vi "SW_Load_settings_from_previous_experiments.vi"(0 "File to load data from":path, 2 "User Name":string="Researcher", 3 "error in (no error)":errorcluster) -> (6 "Settings cluster out":T1, 7 "IO parameters cluster":T2, 9 "Stimulus presets array":T3(array[cluster])=[{"Event type"=0, "Dur., s"=0.0, "Stim., s"=0.0, "Set/Clear"=FALSE, "TTL out N"=1, "Stim. has been set"=FALSE}, {"Event type"=0, "Dur., s"=0.0, "Stim., s"=0.0, "Set/Clear"=FALSE, "TTL out N"=1, "Stim. has been set"=FALSE}, {"Event type"=0, "Dur., s"=0.0, "Stim., s"=0.0, "Set/Clear"=FALSE, "TTL out N"=1, "Stim. has been set"=FALSE}, {"Event type"=0, "Dur., s"=0.0, "Stim., s"=0.0, "Set/Clear"=FALSE, "TTL out N"=1, "Stim. has been set"=FALSE}, {"Event type"=0, "Dur., s"=0.0, "Stim., s"=0.0, "Set/Clear"=FALSE, "TTL out N"=1, "Stim. has been set"=FALSE}, {"Event type"=0, "Dur., s"=0.0, "Stim., s"=0.0, "Set/Clear"=FALSE, "TTL out N"=1, "Stim. has been set"=FALSE}, {"Event type"=0, "Dur., s"=0.0, "Stim., s"=0.0, "Set/Clear"=FALSE, "TTL out N"=1, "Stim. has been set"=FALSE}, {"Event type"=0, "Dur., s"=0.0, "Stim., s"=0.0, "Set/Clear"=FALSE, "TTL out N"=1, "Stim. has been set"=FALSE}, {"Event type"=0, "Dur., s"=0.0, "Stim., s"=0.0, "Set/Clear"=FALSE, "TTL out N"=1, "Stim. has been set"=FALSE}, {"Event type"=0, "Dur., s"=0.0, "Stim., s"=0.0, "Set/Clear"=FALSE, "TTL out N"=1, "Stim. has been set"=FALSE}, {"Event type"=0, "Dur., s"=0.0, "Stim., s"=0.0, "Set/Clear"=FALSE, "TTL out N"=1, "Stim. has been set"=FALSE}, {"Event type"=0, "Dur., s"=0.0, "Stim., s"=0.0, "Set/Clear"=FALSE, "TTL out N"=1, "Stim. has been set"=FALSE}, {"Event type"=0, "Dur., s"=0.0, "Stim., s"=0.0, "Set/Clear"=FALSE, "TTL out N"=1, "Stim. has been set"=FALSE}, {"Event type"=0, "Dur., s"=0.0, "Stim., s"=0.0, "Set/Clear"=FALSE, "TTL out N"=1, "Stim. has been set"=FALSE}] {"Event type" items=["Stay for N seconds"]; "TTL out N" items=["1"=1, "2"=2, "1+2"=3]}, 10 "error out":errorcluster={"status"=TRUE, "code"=1, "source"="Dequeue Element in NI_LVConfig.lvlib:Read Value Without Comment.vi->NI_LVConfig.lvlib:Read Key (I32).vi->SW_Load_settings_to_main_tab.vi"})   [LabVIEW 2016]
uses:
  <vilib>/Utility/config.llb/Config Data RefNum.ctl
  <vilib>/Utility/config.llb/NI_LVConfig.lvlib
panel:
  out "Author's name":string
  out "Settings loaded OK (TDMS)":bool
  out "Data filtering":u16
  out "\"Stop at\" enabled":bool
  out "Name prefix":string
  out "Stop at":dbl
  out "Offset H.":dbl
  out "Twisted neck":bool
  out "Vertical offset":dbl
  out "Bridge swap?":bool
  out "VISA resource name":string
  out "Cage diameter, mm":i32=180
  out "Border segments starting angle":i32
  out "Midfield segments starting angle":i32
  out "Midfield segments outer radius, mm":i32=60
  out "Center segment outer radius, mm":i32=30
  out "Amount of border segments":i32=8
  out "Amount of midfield segments":i32=4
  out "Refnum out":T4
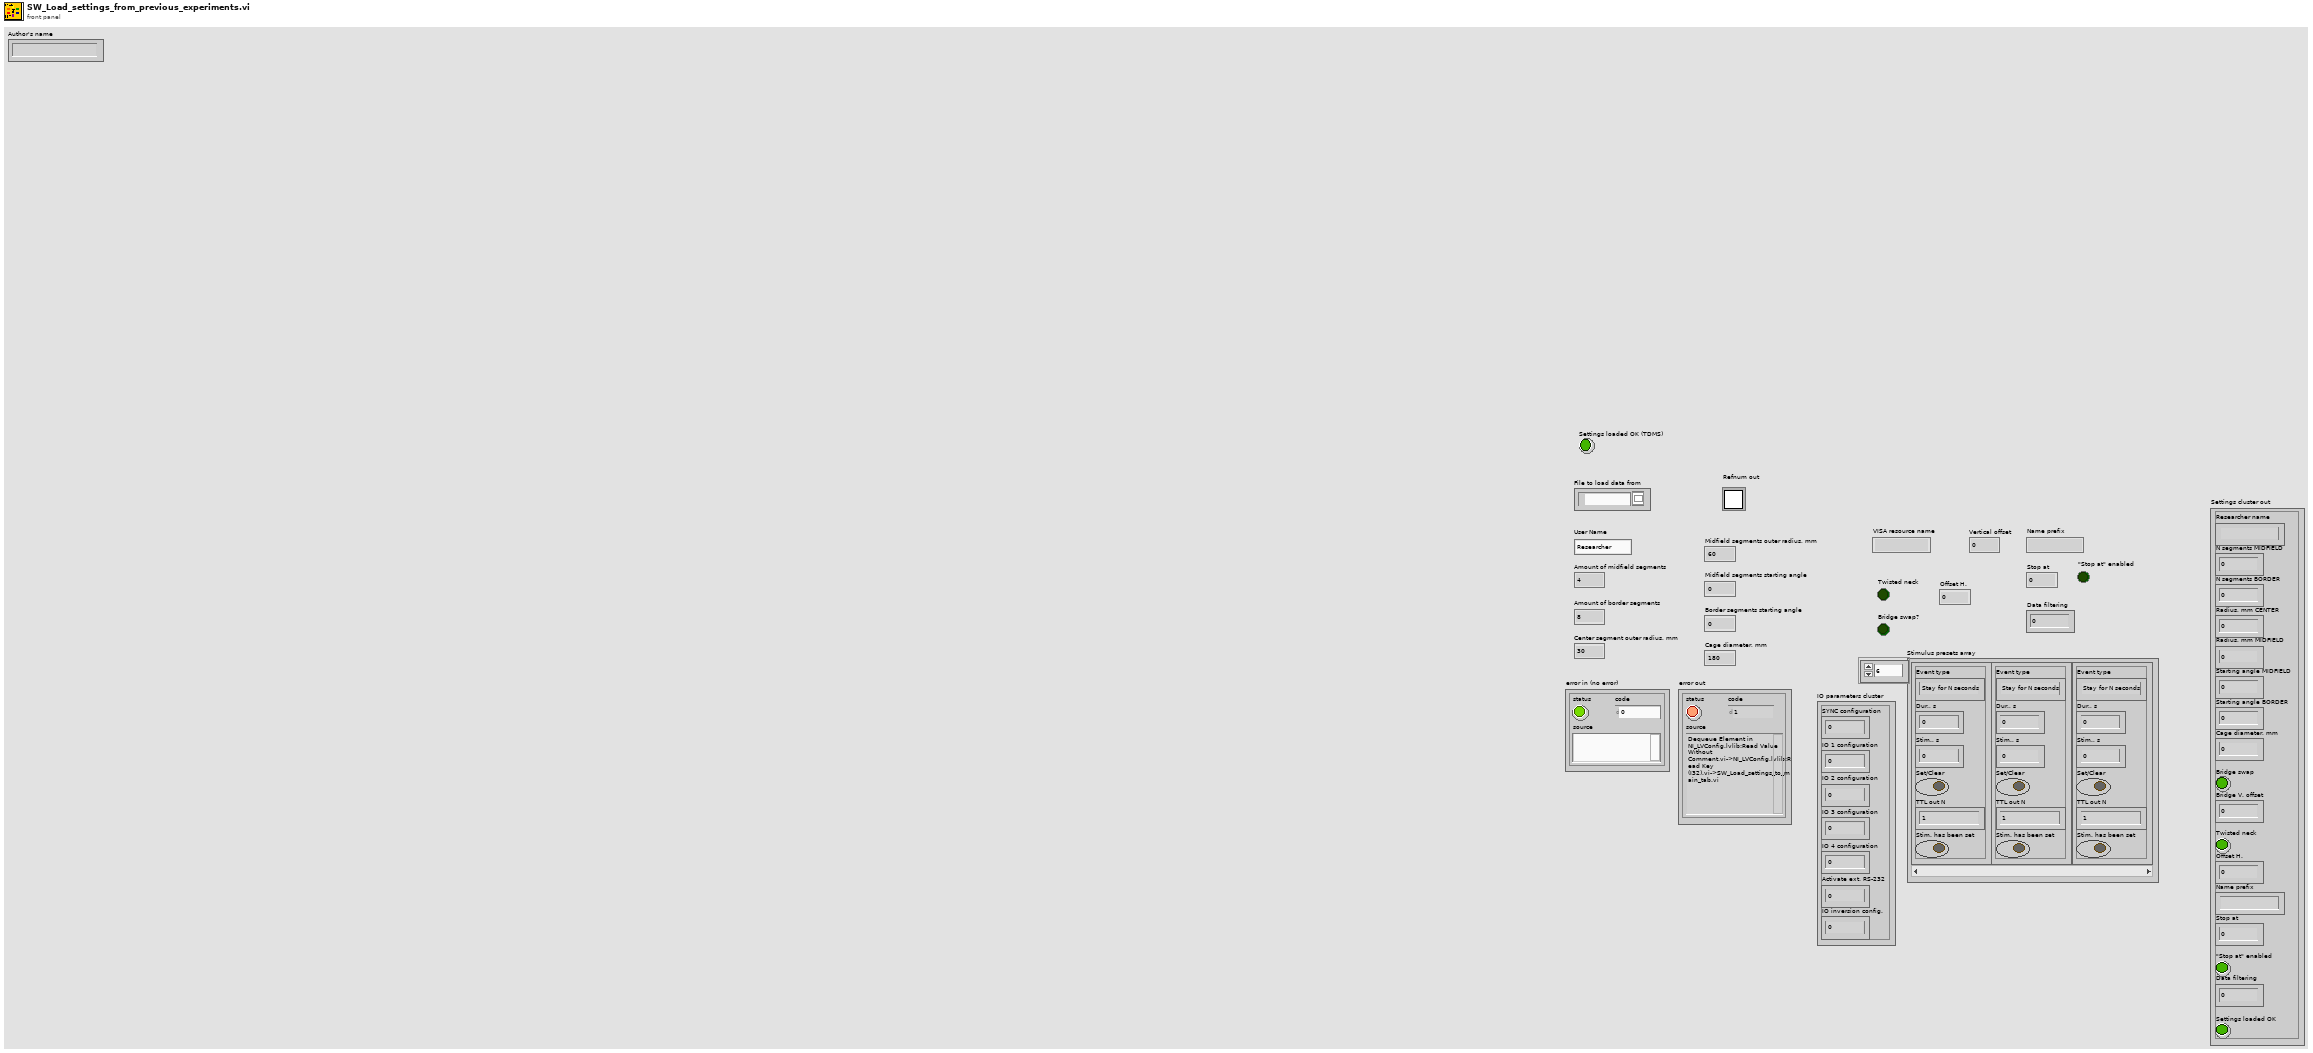
[diagram p1: front panel]
types:
  T1 = cluster{"Researcher name":string, "N segments MIDFIELD":u8, "N segments BORDER":u8, "Radius, mm CENTER":u16, "Radius, mm MIDFIELD":u16, "Starting angle MIDFIELD":i16, "Starting angle BORDER":i16, "Cage diameter, mm":u16, "Bridge swap":bool, "Bridge V. offset":sgl, "Twisted neck":bool, "Offset H.":sgl, "Name prefix":string, "Stop at":dbl, "\"Stop at\" enabled":bool, "Data filtering":u16, "Settings loaded OK":bool}
  T2 = cluster{"SYNC configuration":u16, "IO 1 configuration":u16, "IO 2 configuration":u16, "IO 3 configuration":u16, "IO 4 configuration":u16, "Activate ext. RS-232":u16, "IO inversion config.":u16}
  T3 = cluster{"Event type":u16, "Dur., s":sgl, "Stim., s":sgl, "Set/Clear":bool, "TTL out N":u16, "Stim. has been set":bool}[]
  T4 = typedef "NI_LVConfig.lvlib/Config Data RefNum.ctl" = refnum<k1>
  T5 = cluster{"N segments BORDER":u8, "Starting angle BORDER":i16, "N segments MIDFIELD":u8, "Starting angle MIDFIELD":i16, "Radius, mm MIDFIELD":u16, "Amount of central segments":u8, "Radius, mm CENTER":u16, "Bridge swap":bool, "Bridge V. offset":sgl, "Twisted neck":bool, "Offset H.":sgl, "Zones configuration":string[], "IO parameters string":string, "Cage diameter, mm":u16, "Name prefix":string, "Stop at":dbl, "\"Stop at\" enabled":bool, "Data filtering":u16}
  T6 = enum16{"big-endian, network order", "native, host order", "little-endian"}
  T7 = enum16{"open", "open or create", "create or replace", "create", "open (read-only)"}
  T8 = cluster{"Event type":u16, "Time, s":sgl, "Stimulus, s":sgl, "Set/Clear":bool, "TTL out":u16, "Stim. has been set":bool}
  T9 = cluster{"Event type":u16, "Cond., s":sgl, "Stim., s":sgl, "Set/Clear":bool, "TTL out N":u16, "Stim. has been set":bool}
  T10 = cluster{"array[0]":u16, "array[1]":u16, "array[2]":u16, "array[3]":u16, "array[4]":u16, "array[5]":u16, "array[6]":u16, "array[7]":u16, "array[8]":u16}
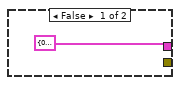
[diagram p2: hidden frame]
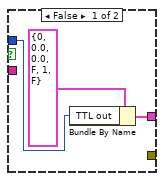
[diagram p10: hidden frame]
diagram:
  n1 = Path To String(path="File to load data from") -> (string=w13:string)
  n2 = To Lower Case(string=w13) -> (all lower case string=w12:string)
  n3 = Reverse String(1:w12) -> (0:w11:string)
  n4 = Search/Split String(string=w11, search string/char (-)=".") -> (substring before match=w9:string)  [unwired: 1 in, 2 out]
  n5 = Reverse String(1:w9) -> (0:w6:string)
  n6 = case shown="\"tdms\", Default" w6 {
    tunnel: [w30 w118] -> w8
    tunnel: [w49 w117] -> w7
    tunnel: "User Name" -> [_ w100]
    tunnel: "File to load data from" -> [w51 w116]
    tunnel: "error in (no error)" -> [w52 w114]
    tunnel: [w50 w112] -> w2
    tunnel: [w14 w111] -> w1
    frame "tdms", Default {
      n7 = TDMS Open(5:FALSE ("create index file? (T)"), 6:TRUE ("disable buffering? (T)"), 7:enum16{"1.0", "2.0"}."2.0" ("file format version (2.0)"), 8:w52, 9:T6."little-endian" ("byte order (2:little-endian)"), 10:T7."open (read-only)" ("operation (0:open)"), 11:w51) -> (0:w66:errorcluster, 3:w67:refnum<k34>)
      n8 = TDMS Get Properties(5:"", 7:"Description" ("property name"), 8:w66, 11:w67) -> (0:w62:errorcluster, 3:w61:refnum<k34>, 4:w63:string, 6:w56:bool)  [unwired: 2 in, 2 out]
      n9 = Unflatten From JSON(JSON string=w63, type and defaults=T5 {"N segments BORDER"=0, "Starting angle BORDER"=0, "N segments MIDFIELD"=0, "Starting angle MIDFIELD"=0, "Radius, mm MIDFIELD"=0, "Amount of central segments"=0, "Radius, mm CENTER"=0, "Bridge swap"=FALSE, "Bridge V. offset"=0.0, "Twisted neck"=FALSE, "Offset H."=0.0, "Zones configuration"=[], "IO parameters string"="[12,1,1,0,0,0]", "Cage diameter, mm"=180, "Name prefix"="SavedTrack", "Stop at"=0.0, "\"Stop at\" enabled"=FALSE, "Data filtering"=5} ("Parameters"), error in (no error)=w62) -> (value=w57:T5, error out=w58:errorcluster)  [unwired: 4 in]
      n10 = TDMS Get Properties(5:"", 7:"Author" ("property name"), 8:w58, 11:w61) -> (0:w27:errorcluster, 4:w47:string, 6:w55:bool)  [unwired: 2 in, 3 out]
      "Author's name" <- w47
      n11 = Unbundle By Name(w57) -> ("N segments MIDFIELD"=w46:u8, "N segments BORDER"=w44:u8, "Radius, mm CENTER"=w43:u16, "Radius, mm MIDFIELD"=w42:u16, "Starting angle MIDFIELD"=w41:i16, "Starting angle BORDER"=w40:i16, "Bridge V. offset"=w37:sgl, "Bridge swap"=w38:bool, "Cage diameter, mm"=w39:u16, "Zones configuration"=w54:string[], "Twisted neck"=w36:bool, "Offset H."=w35:sgl, "Name prefix"=w34:string, "Stop at"=w33:dbl, "\"Stop at\" enabled"=w32:bool, "Data filtering"=w31:u16, "IO parameters string"=w28:string)
      n12 = And(x=w56, y=w55) -> (x .and. y?=w45:bool)
      "Settings loaded OK (TDMS)" <- w45
      n13 = Bundle By Name(cluster=T1 {"Researcher name"="Researcher", "N segments MIDFIELD"=3, "N segments BORDER"=7, "Radius, mm CENTER"=30, "Radius, mm MIDFIELD"=75, "Starting angle MIDFIELD"=0, "Starting angle BORDER"=0, "Cage diameter, mm"=180, "Bridge swap"=FALSE, "Bridge V. offset"=0.0, "Twisted neck"=FALSE, "Offset H."=0.0, "Name prefix"="SavedTrack", "Stop at"=0.0, "\"Stop at\" enabled"=FALSE, "Data filtering"=5, "Settings loaded OK"=FALSE} ("Settings cluster out"), "Researcher name"=w47, "N segments MIDFIELD"=w46, "N segments BORDER"=w44, "Radius, mm CENTER"=w43, "Radius, mm MIDFIELD"=w42, "Starting angle MIDFIELD"=w41, "Starting angle BORDER"=w40, "Cage diameter, mm"=w39, "Bridge swap"=w38, "Bridge V. offset"=w37, "Twisted neck"=w36, "Offset H."=w35, "Name prefix"=w34, "Stop at"=w33, "\"Stop at\" enabled"=w32, "Data filtering"=w31, "Settings loaded OK"=w45) -> (w30:T1)
      n14 = Unflatten From JSON(JSON string=w28, type and defaults=u16[] [] ("array"), error in (no error)=w27) -> (value=w15:u16[], error out=w26:errorcluster)  [unwired: 4 in]
      n15 = Array To Cluster(array=w15) -> (cluster=w23:T10)
      n16 = Unbundle(w23) -> ("array[0]"=w22:u16, "array[1]"=w21:u16, "array[2]"=w20:u16, "array[3]"=w19:u16, "array[4]"=w18:u16, "array[5]"=w17:u16, "array[6]"=w16:u16)  [unwired: 2 out]
      n17 = Bundle By Name(cluster=T2 {"SYNC configuration"=12, "IO 1 configuration"=1, "IO 2 configuration"=1, "IO 3 configuration"=0, "IO 4 configuration"=0, "Activate ext. RS-232"=0, "IO inversion config."=0} ("Sync parameters cluster output"), "SYNC configuration"=w22, "IO 1 configuration"=w21, "IO 2 configuration"=w20, "IO 3 configuration"=w19, "IO 4 configuration"=w18, "Activate ext. RS-232"=w17, "IO inversion config."=w16) -> (w14:T2)
      n18 = for {
        N: 14 -> [_]
        tunnel: w26 -> [w77]
        tunnel: [w79] -> w50
        tunnel: [w80] -> w49 mode=indexing
        tunnel: w54 -> [w75]
        i -> [w76]
        n19 = for {
          tunnel: w75 -> [w91] mode=indexing
          tunnel: w76 -> [w85]
          tunnel: [w84] -> w74
          tunnel: [w83] -> w73
          stop <- w84 stop-if-true
          n20 = Search/Split String(string=w91, search string/char (-)=":") -> (substring before match=w89:string, match + rest of string=w82:string)  [unwired: 1 in, 1 out]
          n21 = String Subset(string=w82, offset (0)=2) -> (substring=w83:string)  [unwired: 1 in]
          n22 = Scan From String(format string="%u", input string=w89, initial scan location=u32 4) -> (output 1=w86:u32)  [unwired: 2 in, 3 out]
          n23 = Equal?(x=w85, y=w86) -> (x = y?=w84:bool)
        }
        n24 = case shown="True" w74 {
          tunnel: w73 -> [_ w96]
          tunnel: [T8 {"Event type"=0, "Time, s"=0.0, "Stimulus, s"=0.0, "Set/Clear"=FALSE, "TTL out"=1, "Stim. has been set"=FALSE} ("Cluster of the stimuls settings") w95] -> w80
          tunnel: [_ w94] -> w78
          frame False {
          }
          frame True {
            n25 = Unflatten From JSON(JSON string=w96, type and defaults=T8 {"Event type"=0, "Time, s"=0.0, "Stimulus, s"=0.0, "Set/Clear"=FALSE, "TTL out"=1, "Stim. has been set"=FALSE} ("Cluster of the stimuls settings")) -> (value=w95:T8, error out=w94:errorcluster)  [unwired: 5 in]
          }
        }
        n26 = Merge Errors(w78, w77) -> (w79:errorcluster)
      }
    }
    frame "trset" {
      w109 = "Data filtering" ("key")
      w140 = "\"Stop at\" enabled"
      w149 = "Stop at" ("key")
      w144 = "SavedTrack" ("default value")
      w152 = "Name prefix"
      w162 = "Offset H." ("key")
      w168 = "Twisted neck"
      w201 = "Bridge offset" ("key")
      w209 = "Bridge swap?"
      w218 = "Cage diameter, mm" ("key")
      w229 = "Border segments starting angle" ("key")
      w230 = "Midfield segments starting angle" ("key")
      w242 = "Midfield segments outer radius, mm" ("key")
      w245 = "Center segment outer radius, mm" ("key")
      w251 = "Amount of border segments" ("key")
      w260 = "Amount of midfield segments" ("key")
      n27 = call <vilib>:"Open Config Data.vi"("error in (no error)"=w114, "configuration file path"=w116) -> ("error out"=w113:errorcluster, "refnum"=w115:T4)  [unwired: 7 in, 1 out]
      n28 = call <vilib>:"Read Key (I32).vi"("section"=w100, "error in (no error)"=w113, "default value"=4, "key"=w260, "refnum"=w115) -> ("error out"=w258:errorcluster, "value"=w132:i32, "found?"=w261:bool)  [unwired: 3 in, 1 out]
      "Amount of midfield segments" <- w132
      n29 = case shown="False" w261 {
        tunnel: w100 -> [w428 _]
        tunnel: w115 -> [w429 w431]
        tunnel: w260 -> [w427 _]
        tunnel: w132 -> [w426 _]
        tunnel: w258 -> [w425 w430]
        tunnel: [w424 w430] -> w255
        tunnel: [w423 w431] -> w257
        frame False {
          n30 = call <vilib>:"Write Key (I32).vi"("section"=w428, "error in (no error)"=w425, "value"=w426, "key"=w427, "refnum"=w429) -> ("error out"=w424:errorcluster, "refnum out"=w423:T4)  [unwired: 4 in, 1 out]
        }
        frame True {
        }
      }
      n31 = call <vilib>:"Read Key (I32).vi"("section"=w100, "error in (no error)"=w255, "default value"=8, "key"=w251, "refnum"=w257) -> ("error out"=w252:errorcluster, "value"=w131:i32, "found?"=w253:bool, "refnum out"=w254:T4)  [unwired: 3 in]
      "Amount of border segments" <- w131
      n32 = case shown="False" w253 {
        tunnel: w100 -> [w419 _]
        tunnel: w254 -> [w420 w422]
        tunnel: w251 -> [w418 _]
        tunnel: w131 -> [w417 _]
        tunnel: w252 -> [w416 w421]
        tunnel: [w415 w421] -> w247
        tunnel: [w414 w422] -> w246
        frame False {
          n33 = call <vilib>:"Write Key (I32).vi"("section"=w419, "error in (no error)"=w416, "value"=w417, "key"=w418, "refnum"=w420) -> ("error out"=w415:errorcluster, "refnum out"=w414:T4)  [unwired: 4 in, 1 out]
        }
        frame True {
        }
      }
      n34 = call <vilib>:"Read Key (I32).vi"("section"=w100, "error in (no error)"=w247, "default value"=30, "key"=w245, "refnum"=w246) -> ("error out"=w250:errorcluster, "value"=w130:i32, "found?"=w249:bool, "refnum out"=w248:T4)  [unwired: 3 in]
      "Center segment outer radius, mm" <- w130
      n35 = case shown="False" w249 {
        tunnel: w100 -> [w410 _]
        tunnel: w248 -> [w411 w413]
        tunnel: w245 -> [w409 _]
        tunnel: w130 -> [w408 _]
        tunnel: w250 -> [w407 w412]
        tunnel: [w406 w412] -> w238
        tunnel: [w405 w413] -> w237
        frame False {
          n36 = call <vilib>:"Write Key (I32).vi"("section"=w410, "error in (no error)"=w407, "value"=w408, "key"=w409, "refnum"=w411) -> ("error out"=w406:errorcluster, "refnum out"=w405:T4)  [unwired: 4 in, 1 out]
        }
        frame True {
        }
      }
      n37 = call <vilib>:"Read Key (I32).vi"("section"=w100, "error in (no error)"=w238, "default value"=60, "key"=w242, "refnum"=w237) -> ("error out"=w239:errorcluster, "value"=w129:i32, "found?"=w240:bool, "refnum out"=w241:T4)  [unwired: 3 in]
      "Midfield segments outer radius, mm" <- w129
      n38 = case shown="False" w240 {
        tunnel: w100 -> [w401 _]
        tunnel: w241 -> [w402 w404]
        tunnel: w242 -> [w400 _]
        tunnel: w129 -> [w399 _]
        tunnel: w239 -> [w398 w403]
        tunnel: [w397 w403] -> w232
        tunnel: [w396 w404] -> w231
        frame False {
          n39 = call <vilib>:"Write Key (I32).vi"("section"=w401, "error in (no error)"=w398, "value"=w399, "key"=w400, "refnum"=w402) -> ("error out"=w397:errorcluster, "refnum out"=w396:T4)  [unwired: 4 in, 1 out]
        }
        frame True {
        }
      }
      n40 = call <vilib>:"Read Key (I32).vi"("section"=w100, "error in (no error)"=w232, "default value"=-90, "key"=w230, "refnum"=w231) -> ("error out"=w236:errorcluster, "value"=w128:i32, "found?"=w235:bool, "refnum out"=w234:T4)  [unwired: 3 in]
      "Midfield segments starting angle" <- w128
      n41 = case shown="False" w235 {
        tunnel: w100 -> [w392 _]
        tunnel: w234 -> [w393 w395]
        tunnel: w230 -> [w391 _]
        tunnel: w128 -> [w390 _]
        tunnel: w236 -> [w389 w394]
        tunnel: [w388 w394] -> w223
        tunnel: [w387 w395] -> w224
        frame False {
          n42 = call <vilib>:"Write Key (I32).vi"("section"=w392, "error in (no error)"=w389, "value"=w390, "key"=w391, "refnum"=w393) -> ("error out"=w388:errorcluster, "refnum out"=w387:T4)  [unwired: 4 in, 1 out]
        }
        frame True {
        }
      }
      n43 = call <vilib>:"Read Key (I32).vi"("section"=w100, "error in (no error)"=w223, "default value"=90, "key"=w229, "refnum"=w224) -> ("error out"=w225:errorcluster, "value"=w127:i32, "found?"=w226:bool, "refnum out"=w227:T4)  [unwired: 3 in]
      "Border segments starting angle" <- w127
      n44 = case shown="False" w226 {
        tunnel: w100 -> [w383 _]
        tunnel: w227 -> [w384 w386]
        tunnel: w229 -> [w382 _]
        tunnel: w127 -> [w381 _]
        tunnel: w225 -> [w380 w385]
        tunnel: [w379 w385] -> w216
        tunnel: [w378 w386] -> w217
        frame False {
          n45 = call <vilib>:"Write Key (I32).vi"("section"=w383, "error in (no error)"=w380, "value"=w381, "key"=w382, "refnum"=w384) -> ("error out"=w379:errorcluster, "refnum out"=w378:T4)  [unwired: 4 in, 1 out]
        }
        frame True {
        }
      }
      n46 = call <vilib>:"Read Key (I32).vi"("section"=w100, "error in (no error)"=w216, "default value"=180, "key"=w218, "refnum"=w217) -> ("error out"=w222:errorcluster, "value"=w126:i32, "found?"=w221:bool, "refnum out"=w220:T4)  [unwired: 3 in]
      "Cage diameter, mm" <- w126
      n47 = case shown="False" w221 {
        tunnel: w100 -> [w374 _]
        tunnel: w220 -> [w375 w377]
        tunnel: w218 -> [w373 _]
        tunnel: w126 -> [w372 _]
        tunnel: w222 -> [w371 w376]
        tunnel: [w370 w376] -> w104
        tunnel: [w369 w377] -> w102
        frame False {
          n48 = call <vilib>:"Write Key (I32).vi"("section"=w374, "error in (no error)"=w371, "value"=w372, "key"=w373, "refnum"=w375) -> ("error out"=w370:errorcluster, "refnum out"=w369:T4)  [unwired: 4 in, 1 out]
        }
        frame True {
        }
      }
      n49 = call <vilib>:"Read Key (U32).vi"("section"=w100, "error in (no error)"=w104, "default value"=5, "key"=w109, "refnum"=w102) -> ("error out"=w105:errorcluster, "value"=w110:u32, "found?"=w106:bool, "refnum out"=w107:T4)  [unwired: 3 in]
      n50 = To Unsigned Word Integer(number=w110) -> (unsigned 16bit integer=w97:u16)
      "Data filtering" <- w97
      n51 = case shown="False" w106 {
        tunnel: w100 -> [w267 _]
        tunnel: w107 -> [w268 w270]
        tunnel: w109 -> [w266 _]
        tunnel: w97 -> [w265 _]
        tunnel: w105 -> [w264 w269]
        tunnel: [w263 w269] -> w103
        tunnel: [w262 w270] -> w101
        frame False {
          n52 = call <vilib>:"Write Key (U32).vi"("section"=w267, "error in (no error)"=w264, "value"=w265, "key"=w266, "refnum"=w268) -> ("error out"=w263:errorcluster, "refnum out"=w262:T4)  [unwired: 4 in, 1 out]
        }
        frame True {
        }
      }
      n53 = call <vilib>:"Read Key (String).vi"("section"="Defaults", "error in (no error)"=w103, "key"="VISA Resource Name", "refnum"=w101) -> ("error out"=w183:errorcluster, "value"=→"VISA resource name":string, "refnum out"=w182:T4)  [unwired: 4 in, 1 out]
      n54 = call <vilib>:"Read Key (Double).vi"("section"=w100, "error in (no error)"=w183, "default value"=0.0, "key"=w201, "refnum"=w182) -> ("error out"=w205:errorcluster, "value"=w125:dbl, "found?"=w203:bool, "refnum out"=w202:T4)  [unwired: 3 in]
      "Vertical offset" <- w125
      n55 = case shown="False" w203 {
        tunnel: [w355 w358] -> w206
        tunnel: [w356 w359] -> w207
        tunnel: w205 -> [w357 w359]
        tunnel: w100 -> [w354 _]
        tunnel: w201 -> [w353 _]
        tunnel: w202 -> [w351 w358]
        frame False {
          n56 = call <vilib>:"Write Key (Double).vi"("use system decimal point (T)"=FALSE ("value"), "section"=w354, "error in (no error)"=w357, "value"=0.0, "key"=w353, "refnum"=w351) -> ("error out"=w356:errorcluster, "refnum out"=w355:T4)  [unwired: 3 in, 1 out]
        }
        frame True {
        }
      }
      n57 = call <vilib>:"Read Key (Boolean).vi"("section"=w100, "error in (no error)"=w207, "default value"=FALSE, "key"=w209, "refnum"=w206) -> ("error out"=w211:errorcluster, "value"=w124:bool, "found?"=w210:bool, "refnum out"=w212:T4)  [unwired: 3 in]
      "Bridge swap?" <- w124
      n58 = case shown="False" w210 {
        tunnel: w212 -> [w364 w368]
        tunnel: [w363 w368] -> w164
        tunnel: [w365 w367] -> w163
        tunnel: w211 -> [w366 w367]
        tunnel: w100 -> [w362 _]
        tunnel: w209 -> [w361 _]
        frame False {
          n59 = call <vilib>:"Write Key (Boolean).vi"("section"=w362, "error in (no error)"=w366, "value"=FALSE, "key"=w361, "refnum"=w364) -> ("error out"=w365:errorcluster, "refnum out"=w363:T4)  [unwired: 4 in, 1 out]
        }
        frame True {
        }
      }
      n60 = call <vilib>:"Read Key (Boolean).vi"("section"=w100, "error in (no error)"=w163, "default value"=FALSE, "key"=w168, "refnum"=w164) -> ("error out"=w166:errorcluster, "value"=w123:bool, "found?"=w167:bool, "refnum out"=w165:T4)  [unwired: 3 in]
      "Twisted neck" <- w123
      n61 = case shown="False" w167 {
        tunnel: w165 -> [w313 w317]
        tunnel: [w312 w317] -> w157
        tunnel: [w314 w316] -> w156
        tunnel: w166 -> [w315 w316]
        tunnel: w100 -> [w311 _]
        tunnel: w168 -> [w310 _]
        frame False {
          n62 = call <vilib>:"Write Key (Boolean).vi"("section"=w311, "error in (no error)"=w315, "value"=FALSE, "key"=w310, "refnum"=w313) -> ("error out"=w314:errorcluster, "refnum out"=w312:T4)  [unwired: 4 in, 1 out]
        }
        frame True {
        }
      }
      n63 = call <vilib>:"Read Key (Double).vi"("section"=w100, "error in (no error)"=w156, "default value"=0.0, "key"=w162, "refnum"=w157) -> ("error out"=w158:errorcluster, "value"=w122:dbl, "found?"=w160:bool, "refnum out"=w161:T4)  [unwired: 3 in]
      "Offset H." <- w122
      n64 = case shown="False" w160 {
        tunnel: [w304 w307] -> w150
        tunnel: [w305 w308] -> w151
        tunnel: w158 -> [w306 w308]
        tunnel: w100 -> [w303 _]
        tunnel: w162 -> [w302 _]
        tunnel: w161 -> [w300 w307]
        frame False {
          n65 = call <vilib>:"Write Key (Double).vi"("use system decimal point (T)"=FALSE ("value"), "section"=w303, "error in (no error)"=w306, "value"=0.0, "key"=w302, "refnum"=w300) -> ("error out"=w305:errorcluster, "refnum out"=w304:T4)  [unwired: 3 in, 1 out]
        }
        frame True {
        }
      }
      n66 = call <vilib>:"Read Key (String).vi"("section"=w100, "error in (no error)"=w151, "default value"=w144, "key"=w152, "refnum"=w150) -> ("error out"=w154:errorcluster, "value"=w121:string, "found?"=w153:bool, "refnum out"=w155:T4)  [unwired: 3 in]
      "Name prefix" <- w121
      n67 = case shown="False" w153 {
        tunnel: w155 -> [w294 w298]
        tunnel: [w293 w298] -> w143
        tunnel: [w295 w297] -> w142
        tunnel: w154 -> [w296 w297]
        tunnel: w100 -> [w292 _]
        tunnel: w152 -> [w291 _]
        tunnel: w144 -> [w290 _]
        frame False {
          n68 = call <vilib>:"Write Key (String).vi"("section"=w292, "error in (no error)"=w296, "value"=w290, "key"=w291, "refnum"=w294) -> ("error out"=w295:errorcluster, "refnum out"=w293:T4)  [unwired: 4 in, 1 out]
        }
        frame True {
        }
      }
      n69 = call <vilib>:"Read Key (Double).vi"("section"=w100, "error in (no error)"=w142, "default value"=0.0, "key"=w149, "refnum"=w143) -> ("error out"=w145:errorcluster, "value"=w120:dbl, "found?"=w147:bool, "refnum out"=w148:T4)  [unwired: 3 in]
      "Stop at" <- w120
      n70 = case shown="False" w147 {
        tunnel: [w285 w288] -> w136
        tunnel: [w286 w289] -> w135
        tunnel: w145 -> [w287 w289]
        tunnel: w100 -> [w284 _]
        tunnel: w149 -> [w283 _]
        tunnel: w148 -> [w281 w288]
        frame False {
          n71 = call <vilib>:"Write Key (Double).vi"("use system decimal point (T)"=FALSE ("value"), "section"=w284, "error in (no error)"=w287, "value"=0.0, "key"=w283, "refnum"=w281) -> ("error out"=w286:errorcluster, "refnum out"=w285:T4)  [unwired: 3 in, 1 out]
        }
        frame True {
        }
      }
      n72 = call <vilib>:"Read Key (Boolean).vi"("section"=w100, "error in (no error)"=w135, "default value"=FALSE, "key"=w140, "refnum"=w136) -> ("error out"=w138:errorcluster, "value"=w119:bool, "found?"=w139:bool, "refnum out"=w137:T4)  [unwired: 3 in]
      "\"Stop at\" enabled" <- w119
      n73 = case shown="False" w139 {
        tunnel: w137 -> [w275 w279]
        tunnel: [w274 w279] -> w134
        tunnel: [w276 w278] -> w133
        tunnel: w138 -> [w277 w278]
        tunnel: w100 -> [w273 _]
        tunnel: w140 -> [w272 _]
        frame False {
          n74 = call <vilib>:"Write Key (Boolean).vi"("section"=w273, "error in (no error)"=w277, "value"=FALSE, "key"=w272, "refnum"=w275) -> ("error out"=w276:errorcluster, "refnum out"=w274:T4)  [unwired: 4 in, 1 out]
        }
        frame True {
        }
      }
      n75 = call <vilib>:"Read Key (String).vi"("section"=w100, "error in (no error)"=w133, "default value"="[12,1,1,0,0,0,0]" ("IO parameters string"), "key"="IO ports configuration", "refnum"=w134) -> ("error out"=w195:errorcluster, "value"=w196:string, "found?"=w199:bool, "refnum out"=w198:T4)  [unwired: 3 in]
      n76 = Unflatten From JSON(JSON string=w196, type and defaults=u16[] [] ("array"), error in (no error)=w195) -> (value=w193:u16[], error out=w194:errorcluster)  [unwired: 4 in]
      n77 = Array To Cluster(array=w193) -> (cluster=w191:T10)
      n78 = case shown="False" w199 {
        tunnel: w198 -> [w345 w349]
        tunnel: [w344 w349] -> w179
        tunnel: [w346 w348] -> w180
        tunnel: w194 -> [w347 w348]
        tunnel: w100 -> [w343 _]
        tunnel: w196 -> [w342 _]
        frame False {
          n79 = call <vilib>:"Read Key (String).vi"("read raw string? (F)"=FALSE ("value"), "section"=w343, "error in (no error)"=w347, "default value"="[12,1,1,0,0,0,0]" ("IO parameters string"), "key"=w342, "refnum"=w345) -> ("error out"=w346:errorcluster, "refnum out"=w344:T4)  [unwired: 2 in, 2 out]
        }
        frame True {
        }
      }
      n80 = Unbundle(w191) -> ("array[0]"=w190:u16, "array[1]"=w189:u16, "array[2]"=w188:u16, "array[3]"=w187:u16, "array[4]"=w186:u16, "array[5]"=w185:u16, "array[6]"=w170:u16)  [unwired: 2 out]
      n81 = Bundle By Name(cluster=T2 {"SYNC configuration"=12, "IO 1 configuration"=1, "IO 2 configuration"=1, "IO 3 configuration"=0, "IO 4 configuration"=0, "Activate ext. RS-232"=0, "IO inversion config."=0} ("Sync parameters cluster output"), "SYNC configuration"=w190, "IO 1 configuration"=w189, "IO 2 configuration"=w188, "IO 3 configuration"=w187, "IO 4 configuration"=w186, "Activate ext. RS-232"=w185, "IO inversion config."=w170) -> (w111:T2)
      n82 = Unbundle By Name(w111) -> ("SYNC configuration"=w177:u16, "IO 1 configuration"=w172:u16, "IO 2 configuration"=w171:u16)
      n83 = call "SW_Gen_Available_TTL_outputs_array.vi"("IO 2 configuration"=w171, "IO 1 configuration"=w172, "SYNC configuration"=w177) -> ("Available TTL outputs array"=w174:cluster{"String":string, "Value":i32}[])
      n84 = Index Array(array=w174, index=0) -> (element=w175:cluster{"String":string, "Value":i32})
      n85 = Bundle By Name(cluster=T1 {"Researcher name"="Researcher", "N segments MIDFIELD"=4, "N segments BORDER"=0, "Radius, mm CENTER"=30, "Radius, mm MIDFIELD"=75, "Starting angle MIDFIELD"=0, "Starting angle BORDER"=0, "Cage diameter, mm"=180, "Bridge swap"=FALSE, "Bridge V. offset"=0.0, "Twisted neck"=FALSE, "Offset H."=0.0, "Name prefix"="SavedTrack", "Stop at"=0.0, "\"Stop at\" enabled"=FALSE, "Data filtering"=5, "Settings loaded OK"=FALSE} ("Settings cluster out"), "Researcher name"=w100, "N segments MIDFIELD"=w132, "N segments BORDER"=w131, "Radius, mm CENTER"=w130, "Radius, mm MIDFIELD"=w129, "Starting angle MIDFIELD"=w128, "Starting angle BORDER"=w127, "Cage diameter, mm"=w126, "Bridge swap"=w124, "Bridge V. offset"=w125, "Twisted neck"=w123, "Offset H."=w122, "Name prefix"=w121, "Stop at"=w120, "\"Stop at\" enabled"=w119, "Data filtering"=w97, "Settings loaded OK"=TRUE) -> (w118:T1)
      n86 = Unbundle By Name(w175) -> ("Value"=w173:i32)
      n87 = for {
        N: 14 -> [_]
        tunnel: w179 -> [w330]
        tunnel: [w329] -> w178
        tunnel: w100 -> [w328]
        tunnel: w180 -> [w326]
        tunnel: [w320] -> w112
        tunnel: [w323] -> w117 mode=indexing
        tunnel: w173 -> [w318]
        i -> [w321]
        n88 = Format Value(string ("")="Zone ", format string="%02d", value (0)=w321) -> (output string=w327:string)
        n89 = call <vilib>:"Read Key (String).vi"("section"=w328, "error in (no error)"=w326, "key"=w327, "refnum"=w330) -> ("error out"=w325:errorcluster, "value"=w324:string, "found?"=w322:bool, "refnum out"=w329:T4)  [unwired: 4 in]
        n90 = case shown="True" w322 {
          tunnel: w324 -> [_ w339]
          tunnel: [w334 w338] -> w323
          tunnel: [_ w337] -> w319
          tunnel: w318 -> [w333 _]
          frame False {
            n91 = Bundle By Name(cluster=T8 {"Event type"=0, "Time, s"=0.0, "Stimulus, s"=0.0, "Set/Clear"=FALSE, "TTL out"=1, "Stim. has been set"=FALSE} ("Cluster of the stimuls settings"), "TTL out"=w333) -> (w334:T8)
          }
          frame True {
            n92 = Unflatten From JSON(JSON string=w339, type and defaults=T9 {"Event type"=0, "Cond., s"=0.0, "Stim., s"=0.0, "Set/Clear"=FALSE, "TTL out N"=1, "Stim. has been set"=FALSE} ("Cluster of the stimuls settings")) -> (value=w338:T9, error out=w337:errorcluster)  [unwired: 5 in]
          }
        }
        n93 = Merge Errors(w319, w325) -> (w320:errorcluster)
      }
      "Refnum out" <- w178
    }
  }
  "Settings cluster out" <- w8
  "Stimulus presets array" <- w7
  "error out" <- w2
  "IO parameters cluster" <- w1
